vi "LaserCal-mW to V (static).vi"(0 "I-O":cluster{"Voltage":dbl[], "Power":dbl[]}, 5 "Level":dbl, 11 "error in (no error)":errorcluster) -> (4 "Voltage":dbl, 6 "Max Power":dbl, 15 "error out":errorcluster)   [LabVIEW 2020]
uses:
  epl-vi-lib/Utility VIs/Math VIs/interp1.vi
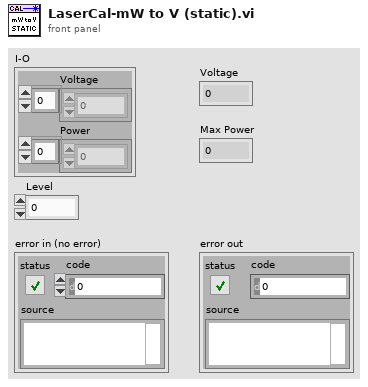
[diagram p1: front panel]
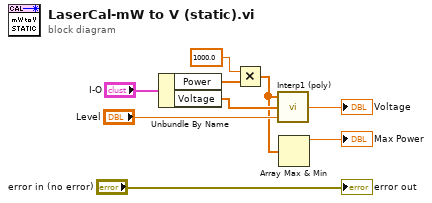
[diagram p0: block diagram]
diagram:
  n1 = Unbundle By Name("I-O") -> ("Power"=w3:dbl[], "Voltage"=w6:dbl[])
  n2 = Multiply(x=1000.0, y=w3) -> (x*y=w1:dbl[])
  n3 = call-poly "Interp1 (poly).vi"("X"=w1, "Y"=w6, "U"="Level") -> ("V"=→"Voltage":dbl)  [unwired: 2 in]
  n4 = Array Max & Min(array=w1) -> (max value=→"Max Power":dbl)  [unwired: 3 out]
  "error out" <- "error in (no error)"
